vi "Timer data class VI - change enum state.vi"(8 "error in (no error)":errorcluster, 10 "State":T1, 11 "Timer in":refnum<class "Timer.lvclass">) -> (0 "error out":errorcluster, 3 "Timer out":refnum<class "Timer.lvclass">)   [LabVIEW 2010, in "Timer.lvclass"]
uses:
  Timer.lvclass
  Controls/Timing Control.ctl
  Timer.lvclass/Timer.ctl
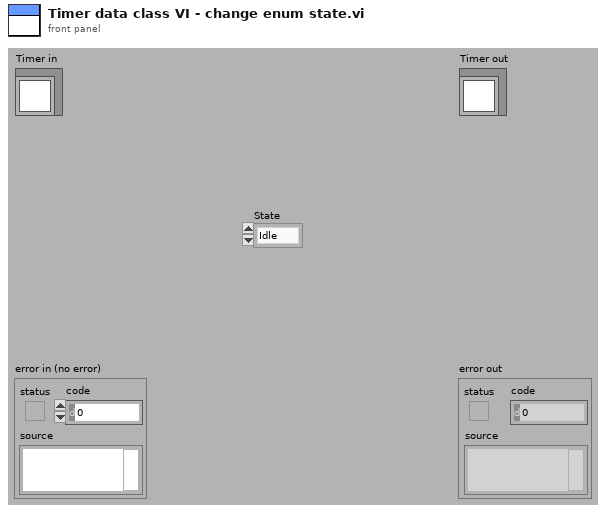
[diagram p1: front panel]
types:
  T1 = typedef "Timing Control.ctl" = enum16{"Idle", "Start", "Continue", "Reset"}
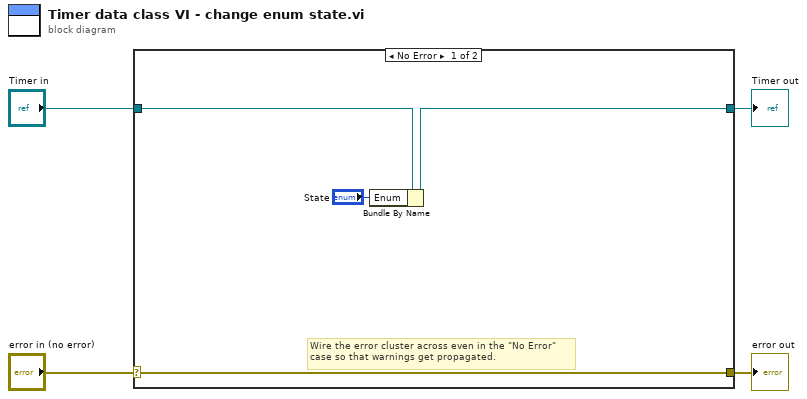
[diagram p0: block diagram]
diagram:
  n1 = case shown="No Error" "error in (no error)" {
    selector: "error in (no error)" -> [w7 w10]
    tunnel: [w7 w10] -> w3
    tunnel: [w6 w9] -> w1
    tunnel: "Timer in" -> [w8 w9]
    frame No Error {
      # "Wire the error cluster across even in the \"No Error\"\ncase so that warnings get propagated."
      n2 = Bundle By Name(cluster=w8, "Enum"="State") -> (w6:refnum<class "Timer.lvclass">)
    }
    frame Error {
    }
  }
  "error out" <- w3
  "Timer out" <- w1
